vi "Format Client Request (Auto-Increment).vi"(8 "error in (no error)":errorcluster, 9 "initial string":string, 10 "JSON Value in":refnum<class "JSON Value.lvclass">, 11 "method":string) -> (0 "error out":errorcluster, 2 "Request String":string)   [LabVIEW 2016, in "JSONRPC Client.lvclass"]
uses:
  JSONRPC Client.lvclass
  <vilib>/NI/JSON Support for LabVIEW/JSON Value/JSON Value.lvclass
  <vilib>/NI/JSON Support for LabVIEW/JSON Value/Object/Insert Value/Insert Value (String).vi
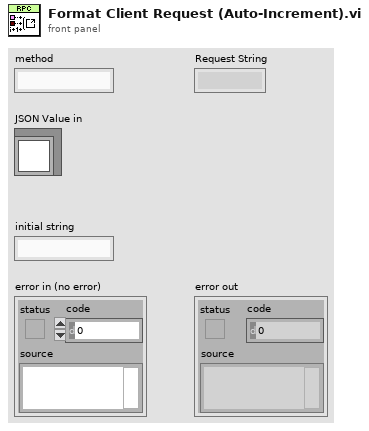
[diagram p1: front panel]
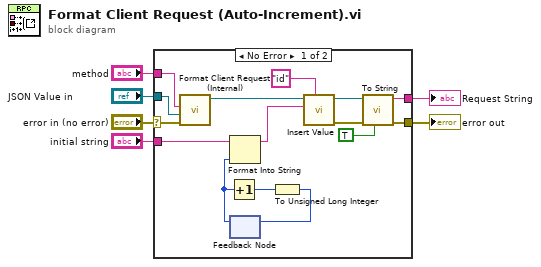
[diagram p0: block diagram]
diagram:
  n1 = case shown="No Error" "error in (no error)" {
    selector: "error in (no error)" -> [w21 w22]
    tunnel: [w8 w22] -> w5
    tunnel: "JSON Value in" -> [w19 _]
    tunnel: "method" -> [w20 _]
    tunnel: "initial string" -> [w18 _]
    tunnel: [w9 _] -> w1
    frame No Error {
      n2 = call "Format Client Request (Internal).vi"("error in (no error)"=w21, "params"=w19, "method"=w20) -> ("JSON Value out"=w12:refnum<class "JSON Value.lvclass">)  [unwired: 7 in, 1 out]
      n3 = feedback #1() -> (w17:u32)  [unwired: 1 in]
      n4 = Increment(x=w17) -> (x+1=w16:u32)
      n5 = Format Into String(initial string=w18, w17) -> (resulting string=w11:string)  [unwired: 2 in, 1 out]
      n6 = To Unsigned Long Integer(number=w16) -> (unsigned 32bit integer=w15:u32)
      n7 = feedback-in #1(w15) -> ()
      n8 = call-poly <vilib>:"Insert Value.vi"("key"="id" ("Name"), "value"=w11, "JSON Value in"=w12) -> ("error out"=w13:errorcluster, "JSON Value out"=w14:refnum<class "JSON Value.lvclass">)  [unwired: 6 in, 1 out]
      n9 = call <vilib>:"To String.vi"("pretty print? (F)"=TRUE ("pretty print? (T)"), "error in (no error)"=w13, "JSON Value in"=w14) -> ("error out"=w8:errorcluster, "String"=w9:string)  [unwired: 7 in]
    }
    frame Error {
    }
  }
  "error out" <- w5
  "Request String" <- w1
